vi "Filter Circles.vi"(1 "Circles":cluster{"x":dbl, "y":dbl, "r":dbl}[](array[cluster])) -> (0 "out":cluster{"x":dbl, "y":dbl, "r":dbl}[](array[cluster]))   [LabVIEW 2018]
panel:
  out "y":dbl
  out "x":dbl
  in  "ok":i32
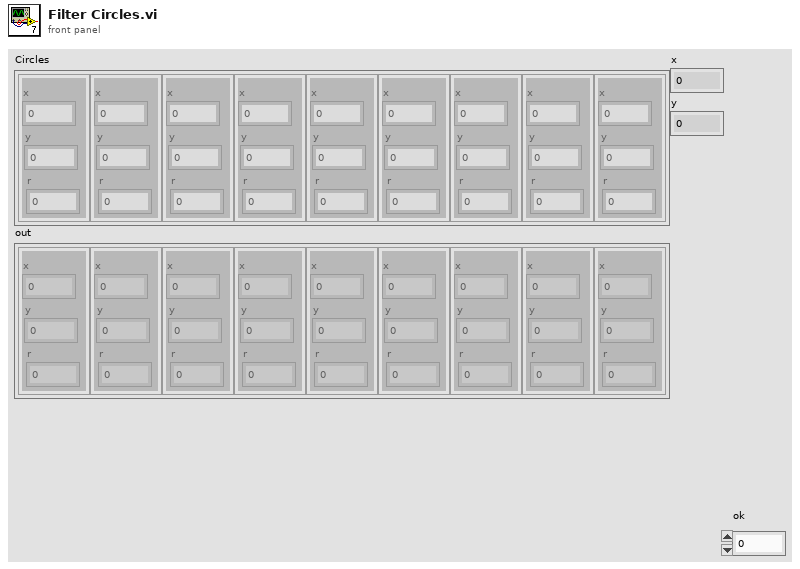
[diagram p1: front panel]
types:
  T1 = cluster{"dimension size":i32, "dimension size":i32, "dimension size":i32}
  T2 = cluster{"dimension size":i32, "dimension size":i32, "dimension size":i32}[]
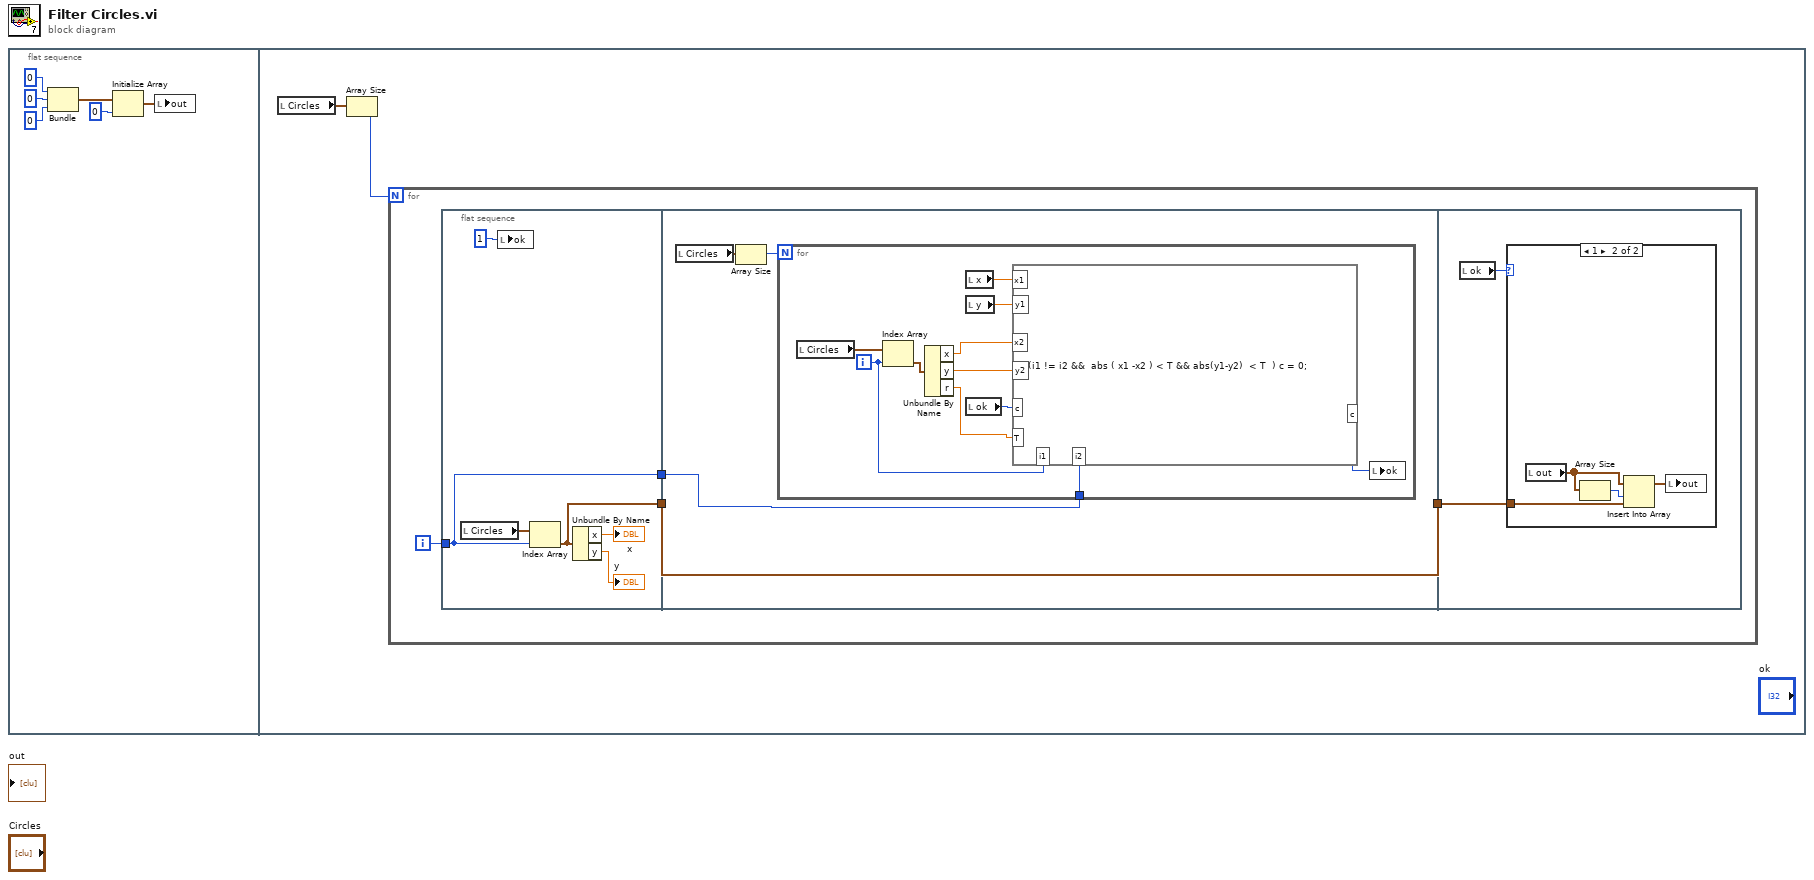
[diagram p0: block diagram]
diagram:
  n1 = flat-sequence {
    frame #0 {
      n2 = Bundle("dimension size"=0, "dimension size"=0, "dimension size"=0) -> (w1:T1)  [unwired: 1 in]
      n3 = Initialize Array(w1, 0 ("dimension size")) -> (w6:T2)
      n4 = local write "out"(w6) -> ()
    }
    frame #1 {
      n5 = local read "Circles"() -> (w8:cluster{"x":dbl, "y":dbl, "r":dbl}[])
      n6 = Array Size(array=w8) -> (size(s)=w7:i32)
      n7 = for {
        N: w7 -> [_]
        i -> [w12]
        n8 = flat-sequence {
          tunnel: w12 -> [w13]
          tunnel: [w14] -> w11
          tunnel: [w13] -> w9
          tunnel: w11 -> [w20]
          tunnel: [w20] -> w10
          tunnel: w9 -> [w19]
          tunnel: w10 -> [w34]
          frame #0 {
            n9 = local read "Circles"() -> (w18:cluster{"x":dbl, "y":dbl, "r":dbl}[])
            n10 = local write "ok"(1 ("ok")) -> ()
            n11 = Index Array(array=w18, index=w13) -> (element=w14:cluster{"x":dbl, "y":dbl, "r":dbl})
            n12 = Unbundle By Name(w14) -> ("x"=→"x":dbl, "y"=→"y":dbl)
          }
          frame #1 {
            n13 = local read "Circles"() -> (w21:cluster{"x":dbl, "y":dbl, "r":dbl}[])
            n14 = Array Size(array=w21) -> (size(s)=w22:i32)
            n15 = for {
              N: w22 -> [_]
              tunnel: w19 -> [w23]
              i -> [w24]
              n16 = local read "Circles"() -> (w33:cluster{"x":dbl, "y":dbl, "r":dbl}[])
              n17 = Index Array(array=w33, index=w24) -> (element=w32:cluster{"x":dbl, "y":dbl, "r":dbl})
              n18 = Unbundle By Name(w32) -> ("x"=w29:dbl, "y"=w28:dbl, "r"=w25:dbl)
              n19 = local read "x"() -> (w31:dbl)
              n20 = local read "y"() -> (w30:dbl)
              n21 = local read "ok"() -> (w27:i32)
              n22 = formula code="if(i1 != i2 &&  abs ( x1 -x2 ) < T && abs(y1-y2)  < T  ) c = 0;"("x1"=w31, "y1"=w30, "x2"=w29, "y2"=w28, "c"=w27, "T"=w25, "i1"=w24, "i2"=w23) -> ("c"=w26:i32)
              n23 = local write "ok"(w26) -> ()
            }
          }
          frame #2 {
            n24 = local read "ok"() -> (w35:i32)
            n25 = case shown="1" w35 {
              tunnel: w34 -> [_ w38]
              frame 0, Default {
              }
              frame 1 {
                n26 = local read "out"() -> (w37:cluster{"x":dbl, "y":dbl, "r":dbl}[])
                n27 = Array Size(array=w37) -> (size(s)=w39:i32)
                n28 = Insert Into Array(array=w37, index=w39, new element=w38) -> (w36:cluster{"x":dbl, "y":dbl, "r":dbl}[])
                n29 = local write "out"(w36) -> ()
              }
            }
          }
        }
      }
    }
  }
